vi "Read RawData.vi"(8 "error in (no error)":errorcluster, 9 "WCM_max_value":bool, 10 "# of scans":i32, 11 "VIS-NIR_STRESING_NEW in":refnum<class "VIS-NIR_STRESING_NEW.lvclass">) -> (0 "error out":errorcluster, 1 "Channel II":sgl[][](array[numeric]), 2 "Channel I":sgl[][](array[numeric]), 3 "VIS-NIR_STRESING_NEW out":refnum<class "VIS-NIR_STRESING_NEW.lvclass">, 4 "WCM_values":sgl[](array[numeric]))   [LabVIEW 2020, in "VIS-NIR_STRESING_NEW.lvclass"]
uses:
  VIS-NIR_STRESING_NEW.lvclass
  Classes/Detector/Detector.lvclass
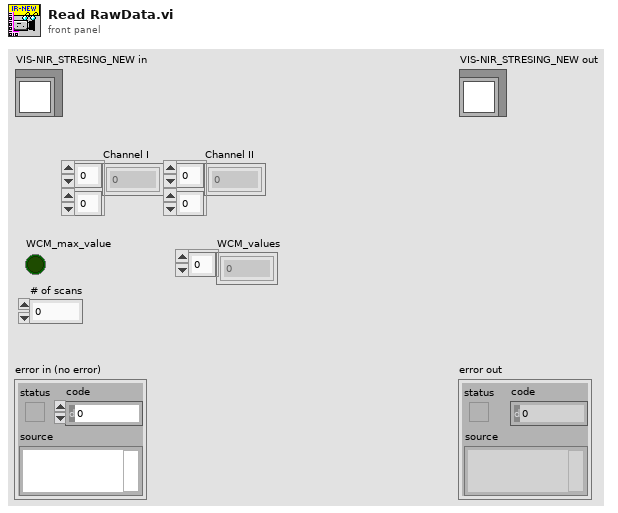
[diagram p1: front panel]
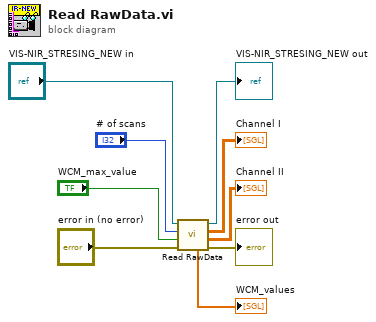
[diagram p0: block diagram]
diagram:
  n1 = call-parent "Read RawData.vi"("error in (no error)"="error in (no error)", "WCM_max_value"="WCM_max_value", "# of scans"="# of scans", "Detector in"="VIS-NIR_STRESING_NEW in") -> ("error out"=→"error out":errorcluster, "Channel II"=→"Channel II":sgl[][], "Channel I"=→"Channel I":sgl[][], "Detector out"=→"VIS-NIR_STRESING_NEW out":refnum<class "VIS-NIR_STRESING_NEW.lvclass">, "WCM_values"=→"WCM_values":sgl[])  [unwired: 3 in]
